vi "DB.vi"(0 "Data":T2={"Identity"=1, "Time"="俞忠达", "Meaning"="你好", "Thumb"=1, "Index"=1, "Middle"=1, "ring"=1, "little"=1, "wrist"=1, "arm"=1, "rota"=1, "delay"=1} {"arm" format="%#.0g"; "ring" format="%#.0g"; "Thumb" format="%#.0g"}, 1 "Beginning State":T5=enum."Inquire All DB" caption="状态", 2 "Delete Num":string[](array[string])=["0", "5"], 3 "Sort As":T3(ring)=enum."时间", 4 "Order":enum32{"Ascend", "Descend"}(radio), 5 "ErrI(No Error)":errorcluster, 6 "Data Table":T4={"Time_Table"="时间", "Meaning"="语义", "Thumb"="拇指", "arm"="手臂", "delay"="延时时间", "Identity"="ID", "passport"="", "Index"="食指", "Middle"="中指", "ring"="无名指", "little"="小手指", "wrist"="手腕", "rota"="转台", "Filename"="PZJData.mdb", "Table"="ACTION_DB"}, 7 "ID Manul？":bool) -> (13 "路径":string="Provider=Microsoft.Jet.OLEDB.4.0;Data Source=D:\\other\\项目\\手语项目\\Data Base\\PZJData.mdb;Persist Security Info=False", 14 "Data_Out":i32(listbox)=-1, 15 "Item Data":string[][](array[string])=[["0", "2017/2/3 20:41:53", "语义", "1", "1", "1", "1", "1", "1", "1", "1", "1"], ["1", "2017/2/3 20:43:36", "语义", "1", "1", "1", "1", "1", "1", "1", "1", "1"], ["2", "2017/2/3 20:51:23", "语义", "1", "1", "1", "1", "1", "1", "1", "1", "1"], ["3", "2017/2/3 20:51:25", "语义", "1", "1", "1", "1", "1", "1", "1", "1", "1"], ["4", "2017/2/3 20:51:26", "语义", "1", "1", "1", "1", "1", "1", "1", "1", "1"], ["5", "2017/2/3 20:51:27", "语义", "1", "1", "1", "1", "1", "1", "1", "1", "1"], ["6", "2017/2/3 20:51:29", "语义", "1", "1", "1", "1", "1", "1", "1", "1", "1"]], 16 "tables":string[](array[string])=["ACTION_DB"], 17 "State Out":string, 18 "New Data":string[](array[string]), 19 "ErrO":errorcluster)   [LabVIEW 2016]
uses:
  StateMachineStates.ctl
  Insertdata.ctl
  <vilib>/addons/database/Auxilliary.llb/DB Tools DataTypes.ctl
  <vilib>/addons/database/Connection.llb/DB Tools Open Connec (String).vi
  <vilib>/addons/database/Connection.llb/Conn Execute.vi
  <vilib>/addons/database/Recordset.llb/Rec Fetch Recordset Data (R).vi
  <vilib>/addons/database/Recordset.llb/Rec Destroy - Connection.vi
  <vilib>/addons/database/_DB Variant To Data/Database Variant To Data.xnode
  <vilib>/addons/database/NI_Database_API.lvlib
panel:
  out "输出簇":T1={"Identity"=6, "Time"="2017/2/3 20:51:29", "Meaning"="语义", "Thumb"=1, "Index"=1, "Middle"=1, "ring"=1, "little"=1, "wrist"=1, "arm"=1, "rota"=1, "delay"=1}
  out "Connection":string="Provider=Microsoft.Jet.OLEDB.4.0;Data Source=D:\\other\\项目\\手语项目\\Data Base\\PZJData.mdb;Persist Security Info=False"
  out "大小":i32[](array[numeric])=[3, 7]
  out "状态":bool
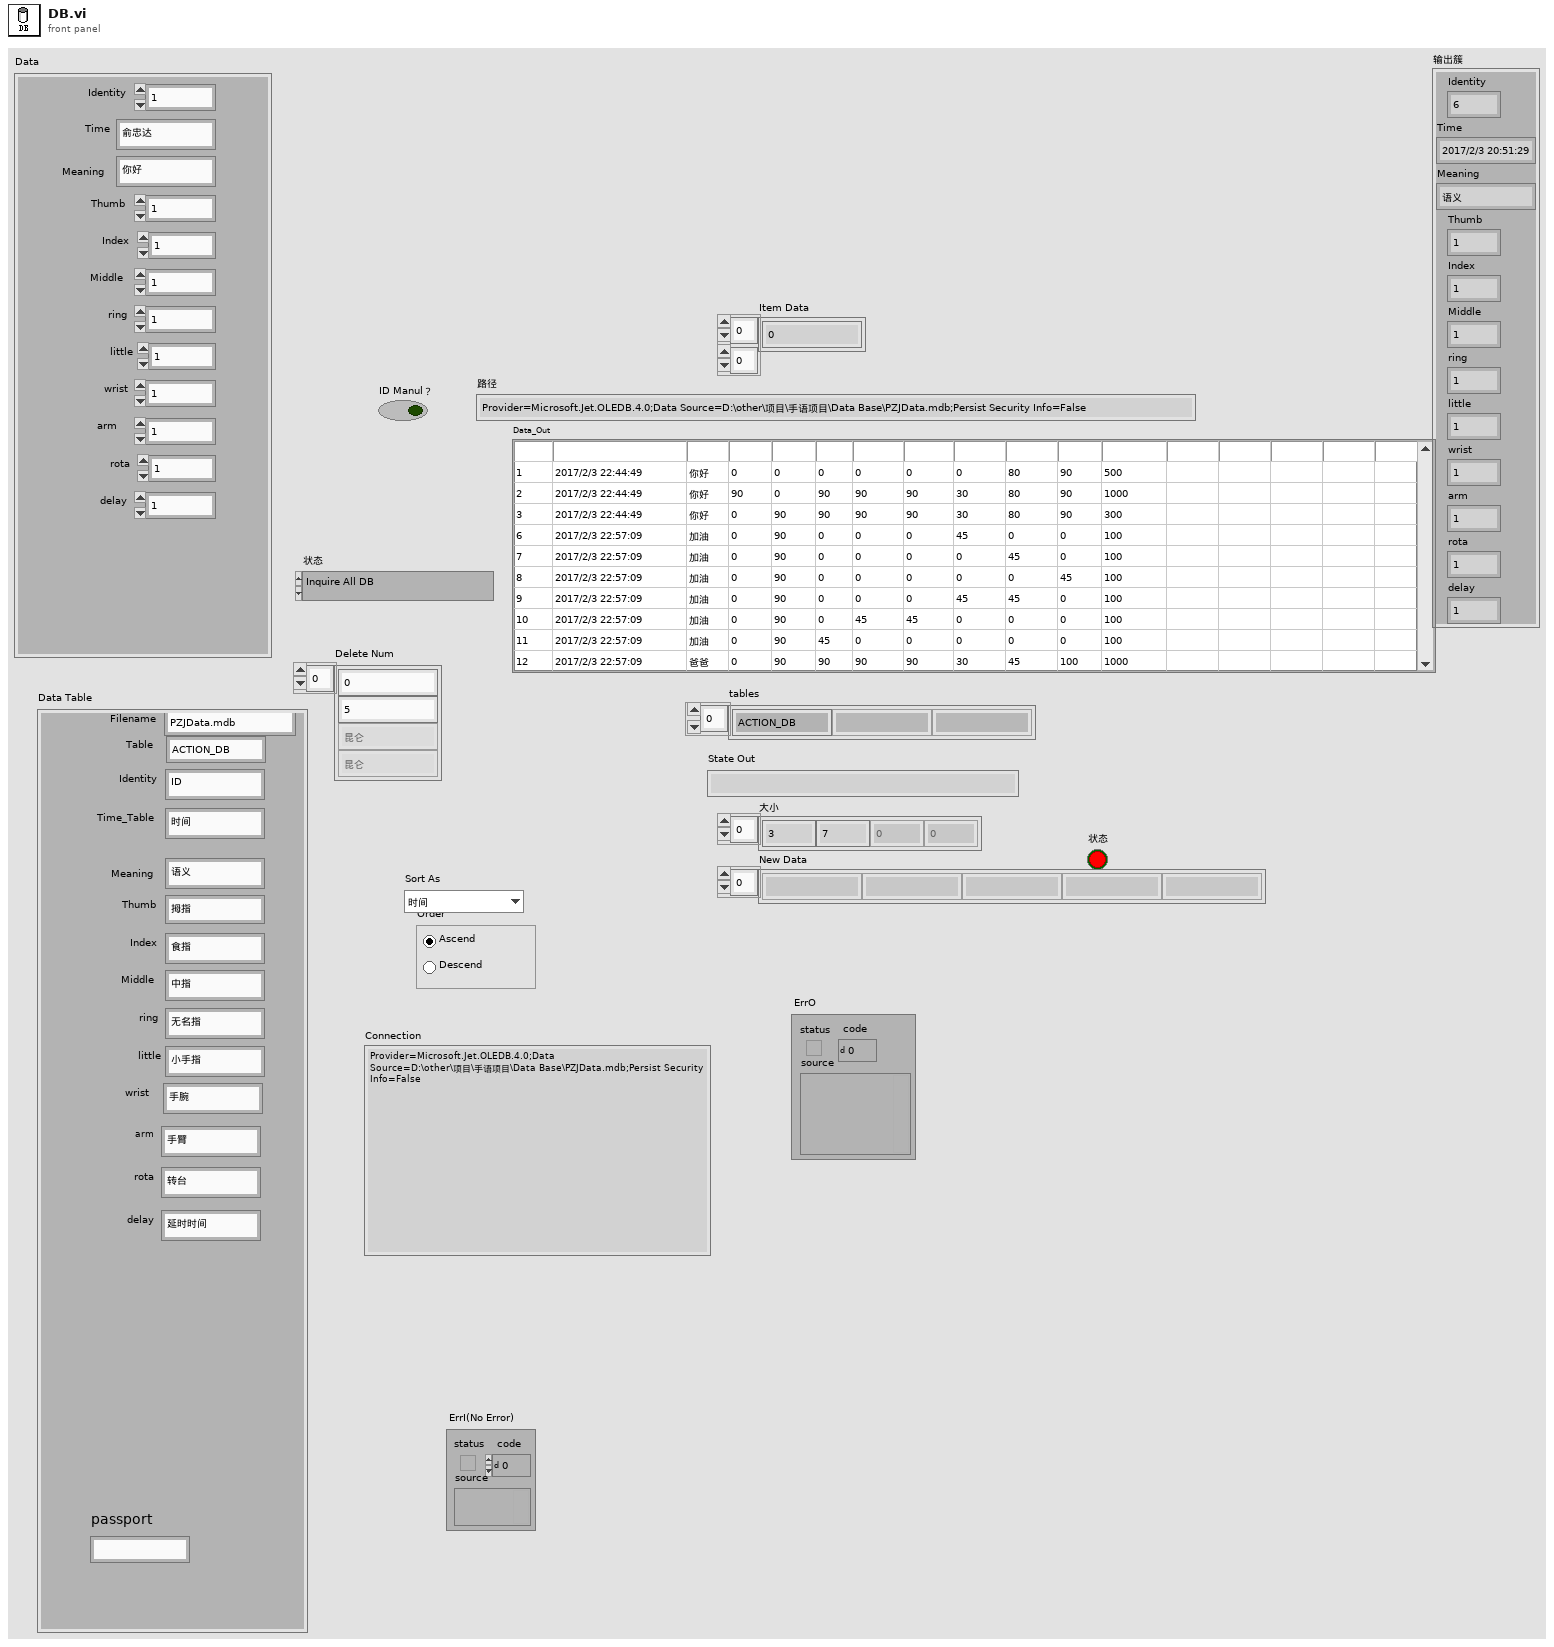
[diagram p1: front panel]
types:
  T1 = cluster{"Identity":i32, "Time":string, "Meaning":string, "Thumb":i32, "Index":i32, "Middle":i32, "ring":i32, "little":i32, "wrist":i32, "arm":i32, "rota":i32, "delay":i32}
  T2 = typedef "Insertdata.ctl" = cluster{"Identity":i32, "Time":string, "Meaning":string, "Thumb":i32, "Index":i32, "Middle":i32, "ring":i32, "little":i32, "wrist":i32, "arm":i32, "rota":i32, "delay":i32}
  T3 = enum16{"ID", "操作者", "级数", "个数", "角度", "时间", "机匣型号", ""}
  T4 = cluster{"Time_Table":string, "Meaning":string, "Thumb":string, "arm":string, "delay":string, "Identity":string, "passport":string, "Index":string, "Middle":string, "ring":string, "little":string, "wrist":string, "rota":string, "Filename":string, "Table":string}
  T5 = typedef "StateMachineStates.ctl" = enum16{"Connection DB", "Creat DB", "Delete Table", "Insert DB", "Inquire Table", "Inquire All DB", "Delete All Data", "Delete Data", "Sort Data", "Inquire Last Data", ""}
  T6 = typedef "NI_Database_API.lvlib/DB Tools DataTypes.ctl" = enum16{"String", "Long (I32)", "Single (SGL)", "Double (DBL)", "Date/Time", "Binary"}
  T7 = typedef "NI_Database_API.lvlib/DB Tools Column Info.ctl" = cluster{"column name":string, "data type":T6, "size":i32, "allow null?":bool}
  T8 = cluster{"Identity":dbl, "Time":string, "Operator":string, "Type":string, "Class":dbl, "Num":dbl, "Angle":dbl}
  T9 = typedef "NI_Database_API.lvlib/Conn ObjectReference.ctl" = refnum<k1>
  T10 = typedef "NI_Database_API.lvlib/Rec ObjectReference.ctl" = refnum<k1>
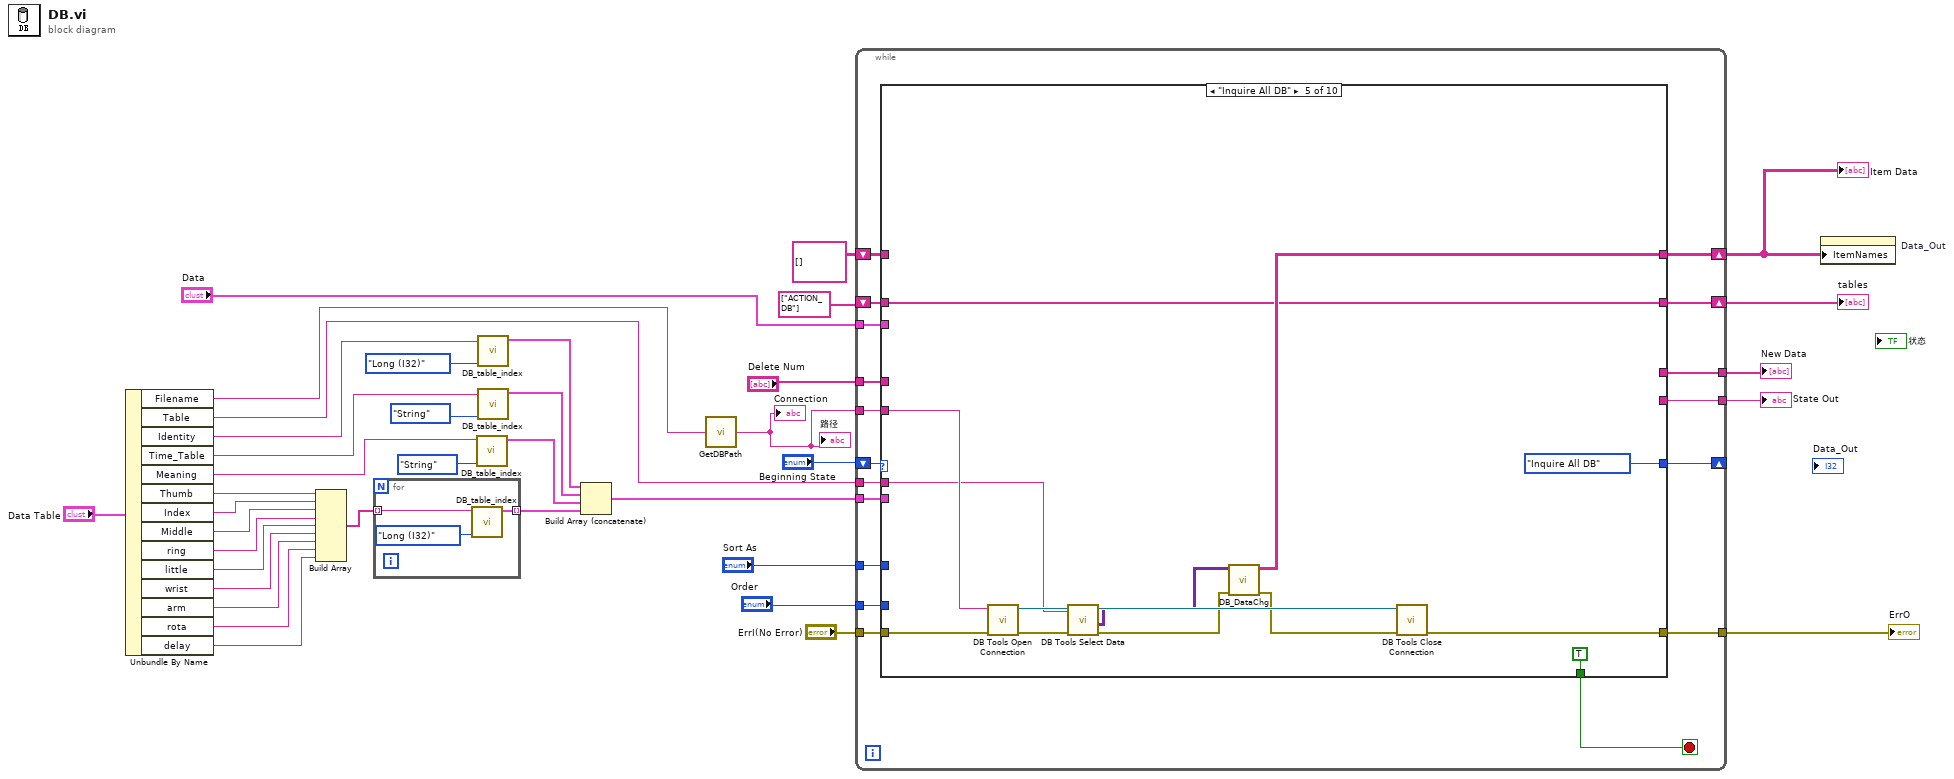
[diagram p0: block diagram]
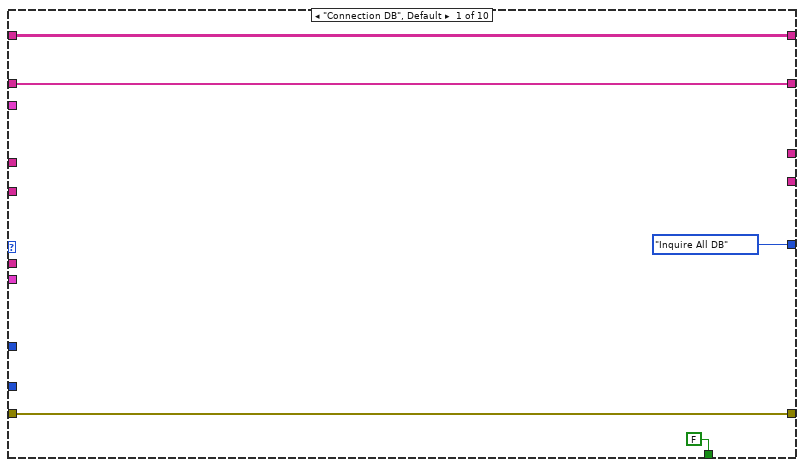
[diagram p2: hidden frame]
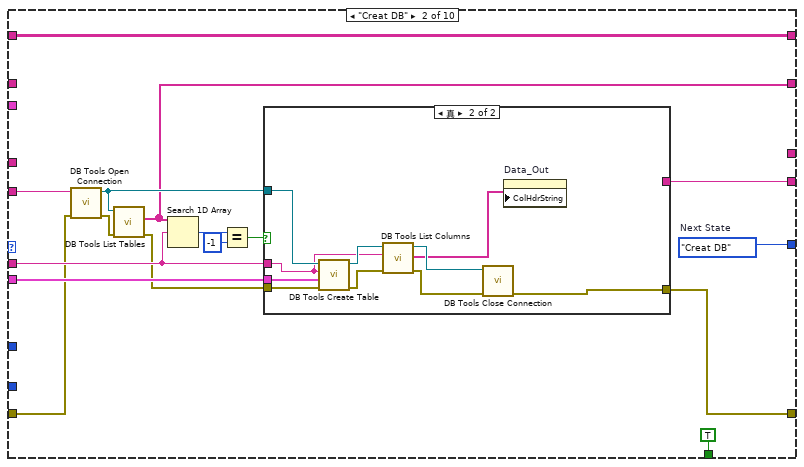
[diagram p3: hidden frame]
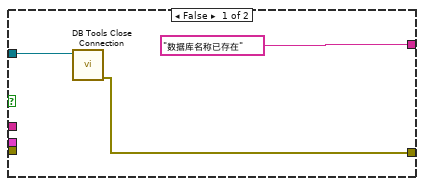
[diagram p4: hidden frame]
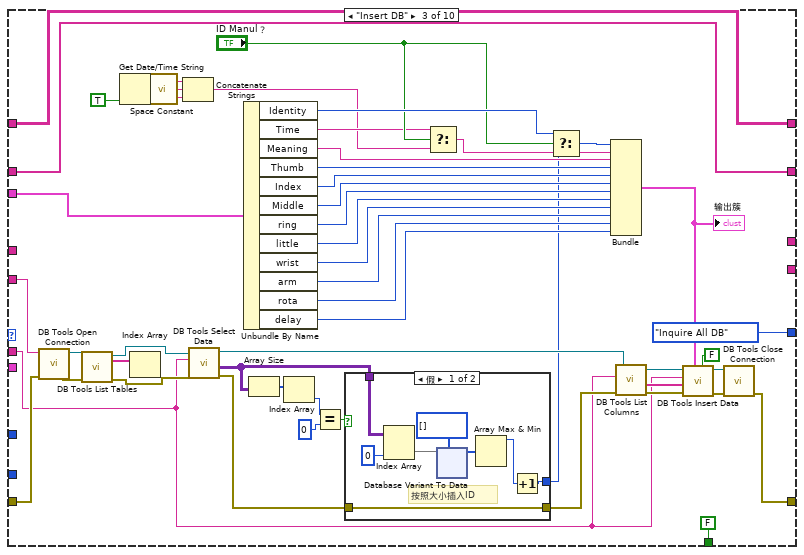
[diagram p5: hidden frame]
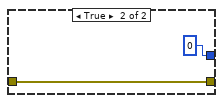
[diagram p6: hidden frame]
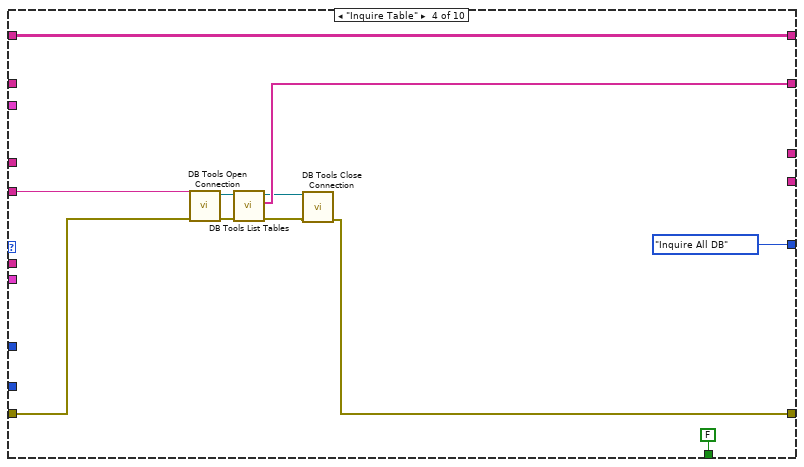
[diagram p7: hidden frame]
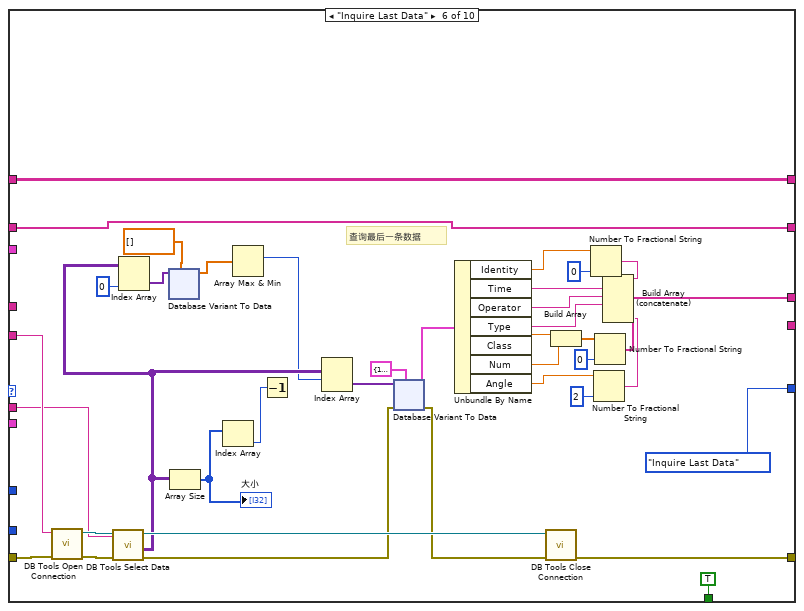
[diagram p8: hidden frame]
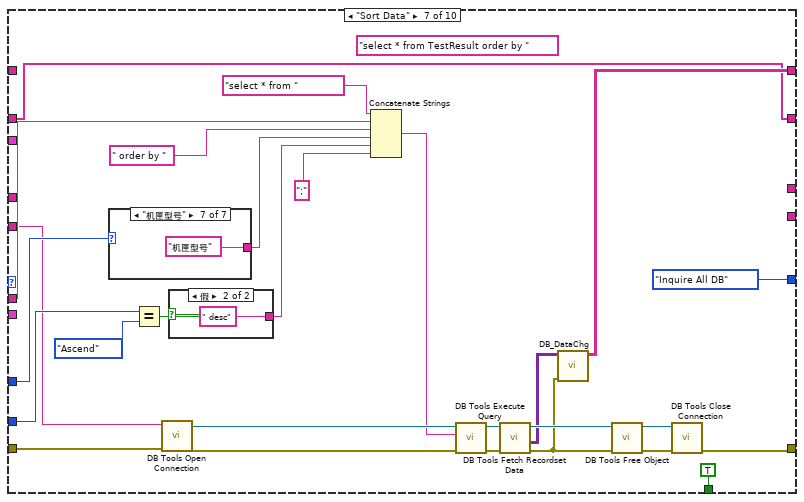
[diagram p9: hidden frame]
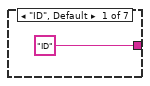
[diagram p10: hidden frame]
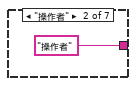
[diagram p11: hidden frame]
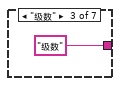
[diagram p12: hidden frame]
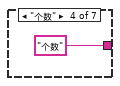
[diagram p13: hidden frame]
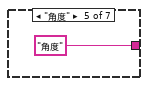
[diagram p14: hidden frame]
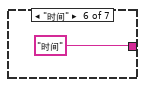
[diagram p15: hidden frame]
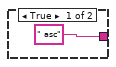
[diagram p16: hidden frame]
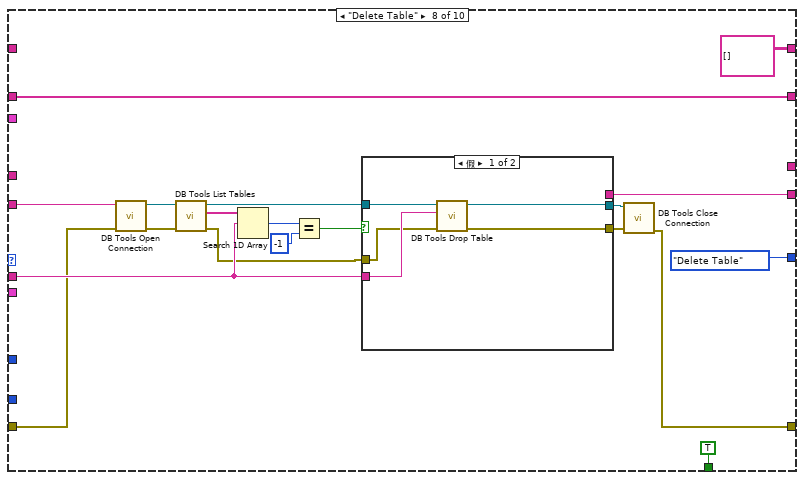
[diagram p17: hidden frame]
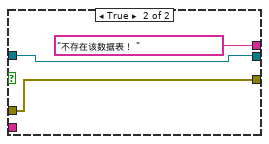
[diagram p18: hidden frame]
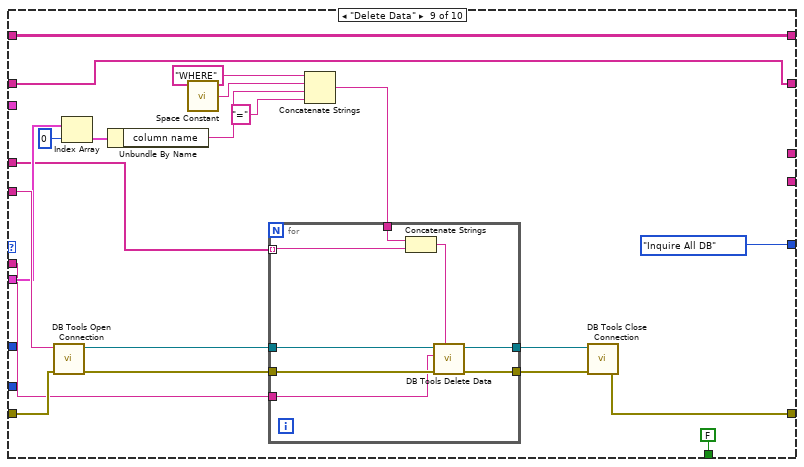
[diagram p19: hidden frame]
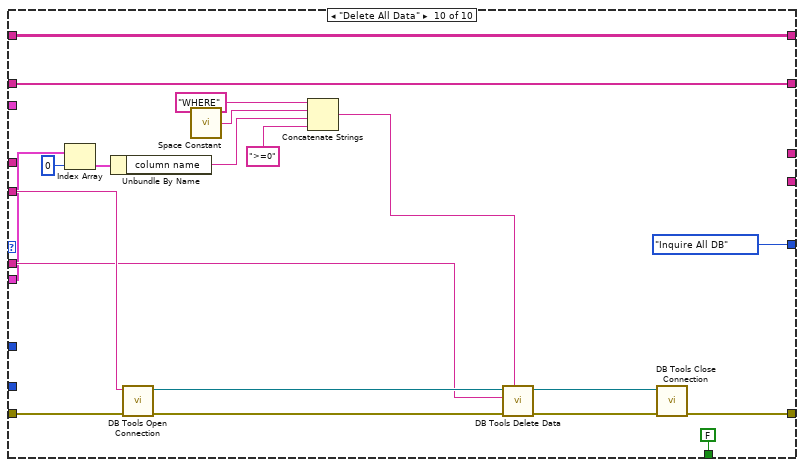
[diagram p20: hidden frame]
diagram:
  n1 = Unbundle By Name("Data Table") -> ("Filename"=w25:string, "Table"=w24:string, "Identity"=w21:string, "Time_Table"=w18:string, "Meaning"=w15:string, "Thumb"=w10:string, "Index"=w9:string, "Middle"=w8:string, "ring"=w7:string, "little"=w6:string, "wrist"=w5:string, "arm"=w4:string, "rota"=w3:string, "delay"=w2:string)
  n2 = Build Array(w10, w9, w8, w7, w6, w5, w4, w3, w2) -> (w1:string[])
  n3 = for {
    tunnel: [w41] -> w36 mode=indexing
    tunnel: w1 -> [w39] mode=indexing
    n4 = call "DB_table_index.vi"("data type"=DB_Tools_DataTypes."Long (I32)", "Thumb"=w39) -> ("column information 2"=w41:T7)  [unwired: 9 in]
  }
  n5 = call "DB_table_index.vi"("data type"=DB_Tools_DataTypes."String", "Thumb"=w15) -> ("column information 2"=w14:T7)  [unwired: 9 in]
  n6 = call "DB_table_index.vi"("data type"=DB_Tools_DataTypes."Long (I32)", "Thumb"=w21) -> ("column information 2"=w20:T7)  [unwired: 9 in]
  n7 = call "DB_table_index.vi"("data type"=DB_Tools_DataTypes."String", "Thumb"=w18) -> ("column information 2"=w16:T7)  [unwired: 9 in]
  n8 = Build Array (concatenate)(w20, w16, w14, w36) -> (w37:T7[])
  n9 = call "GetDBPath.vi"("Filename"=w25) -> ("Connection"=w23:string)
  "Connection" <- w23
  "路径" <- w23
  n10 = while {
    shift-right: [w58] -> _
    shift-left: "Beginning State" -> [w59]
    tunnel: w37 -> [w57]
    tunnel: w24 -> [w56]
    tunnel: w23 -> [w55]
    tunnel: [w54] -> w35
    tunnel: "ErrI(No Error)" -> [w52]
    tunnel: [w51] -> w32
    tunnel: "Data" -> [w50]
    shift-right: [w49] -> w30
    shift-left: string[][] [] -> [w48]
    tunnel: "Delete Num" -> [w46]
    tunnel: "Sort As" -> [w45]
    tunnel: "Order" -> [w44]
    tunnel: [w43] -> w22
    shift-right: [w53] -> w34
    shift-left: string[] ["ACTION_DB"] ("tables 2") -> [w42]
    stop <- w47 stop-if-true
    n11 = case shown="\"Inquire All DB\"" w59 {
      tunnel: [StateMachineStates."Inquire All DB" ("Next State") w80 StateMachineStates."Inquire All DB" ("Next State") StateMachineStates."Inquire All DB" ("Next State") StateMachineStates."Inquire All DB" ("Next State") StateMachineStates."Inquire Last Data" ("Next State") StateMachineStates."Inquire All DB" ("Next State") StateMachineStates."Delete Table" ("Next State") StateMachineStates."Inquire All DB" ("Next State") StateMachineStates."Inquire All DB" ("Next State")] -> w58
      tunnel: w57 -> [_ w73 _ _ _ _ _ _ w594 w609]
      tunnel: w56 -> [_ w72 w94 _ w212 w251 w531 w562 w587 w619]
      tunnel: w55 -> [_ w79 w143 w201 w216 w252 w521 w568 w596 w622]
      tunnel: [_ w74 _ _ _ _ _ w560 _ _] -> w54
      tunnel: [w60 w71 w96 w198 w203 w217 w515 w551 w578 w607] -> w53
      tunnel: w52 -> [w64 w66 w142 w200 w215 w228 w523 w554 w595 w623]
      tunnel: [w64 w70 w136 w195 w210 w248 w522 w555 w582 w616] -> w51
      tunnel: w50 -> [_ _ w109 _ _ _ _ _ _ _]
      tunnel: [w63 w69 w108 w194 w208 w247 w516 string[][] [] w579 w624] -> w49
      tunnel: w48 -> [w63 w69 w108 w194 _ w247 _ _ w579 w624]
      tunnel: [FALSE TRUE FALSE FALSE TRUE TRUE TRUE TRUE FALSE FALSE] -> w47
      tunnel: w46 -> [_ _ _ _ _ _ _ _ w580 _]
      tunnel: w45 -> [_ _ _ _ _ _ w535 _ _ _]
      tunnel: w44 -> [_ _ _ _ _ _ w534 _ _ _]
      tunnel: [_ _ _ _ _ w219 _ _ _ _] -> w43
      tunnel: w42 -> [w60 _ w96 _ w203 w217 w515 w551 w578 w607]
      frame "Connection DB", Default {
      }
      frame "Creat DB" {
        w80 = StateMachineStates."Creat DB"  # Next State
        n12 = call-poly <vilib>:"DB Tools Open Connection.vi"("error in (no error)"=w66, "connection information"=w79) -> ("error out"=w67:errorcluster, "connection reference"=w78:T9)  [unwired: 6 in]
        n13 = call <vilib>:"DB Tools List Tables.vi"("error in (no error)"=w67, "connection reference"=w78) -> ("error out"=w65:errorcluster, "tables"=w71:string[])  [unwired: 3 in, 1 out]
        n14 = Search 1D Array(1D array=w71, element=w72) -> (index of element=w77:i32)  [unwired: 1 in]
        n15 = Equal?(x=w77, y=-1) -> (x = y?=w75:bool)
        n16 = case shown="真" w75 {
          tunnel: w78 -> [w82 w93]
          tunnel: ["数据库名称已存在" _] -> w74
          tunnel: w73 -> [_ w92]
          tunnel: w72 -> [_ w87]
          tunnel: [w81 w91] -> w70
          tunnel: w65 -> [_ w90]
          frame False {
            n17 = call <vilib>:"DB Tools Close Connection.vi"("connection reference"=w82) -> ("error out"=w81:errorcluster)  [unwired: 6 in]
          }
          frame True {
            n18 = call <vilib>:"DB Tools Create Table.vi"("error in (no error)"=w90, "column information"=w92, "table"=w87, "connection reference"=w93) -> ("error out"=w85:errorcluster, "connection reference out"=w89:T9)  [unwired: 4 in]
            n19 = call <vilib>:"DB Tools List Columns.vi"("error in (no error)"=w85, "table"=w87, "connection reference"=w89) -> ("error out"=w84:errorcluster, "columns"=w86:string[], "connection reference out"=w88:T9)  [unwired: 1 in, 1 out]
            n20 = call <vilib>:"DB Tools Close Connection.vi"("error in (no error)"=w84, "connection reference"=w88) -> ("error out"=w91:errorcluster)  [unwired: 5 in]
            n21 = property on="Data_Out" class="MCListbox (严格)"("ColHdrString"=w86) -> ()  [unwired: 2 in, 2 out]
          }
        }
      }
      frame "Insert DB" {
        n22 = call-poly <vilib>:"DB Tools Open Connection.vi"("error in (no error)"=w142, "connection information"=w143) -> ("error out"=w101:errorcluster, "connection reference"=w95:T9)  [unwired: 6 in]
        n23 = call <vilib>:"DB Tools List Tables.vi"("error in (no error)"=w101, "connection reference"=w95) -> ("error out"=w99:errorcluster, "tables"=w100:string[], "connection reference out"=w98:T9)  [unwired: 3 in]
        n24 = Get Date/Time String(want seconds? (F)=TRUE) -> (date string=w115:string, time string=w117:string)  [unwired: 2 in]
        n25 = Index Array(array=w100) -> ()  [unwired: 1 in, 1 out]
        n26 = call <vilib>:"Space Constant.vi"() -> ("String"=w116:string)
        n27 = Concatenate Strings(w115, w116, w117) -> (w111:string)
        n28 = call <vilib>:"DB Tools Select Data.vi"("error in (no error)"=w99, "table"=w94, "connection reference"=w98) -> ("error out"=w132:errorcluster, "data"=w120:variant[][], "connection reference out"=w134:T9)  [unwired: 3 in]
        n29 = Unbundle By Name(w109) -> ("Identity"=w118:i32, "Time"=w112:string, "Meaning"=w127:string, "Thumb"=w128:i32, "Index"=w129:i32, "Middle"=w130:i32, "ring"=w131:i32, "little"=w107:i32, "wrist"=w106:i32, "arm"=w105:i32, "rota"=w104:i32, "delay"=w103:i32)
        n30 = Array Size(array=w120) -> (size(s)=w126:i32[])
        n31 = Index Array(array=w126) -> (element=w123:i32)  [unwired: 1 in]
        n32 = Equal?(x=w123, y=0) -> (x = y?=w124:bool)
        n33 = case shown="假" w124 {
          tunnel: [w146 w191] -> w133
          tunnel: w132 -> [w146 w191]
          tunnel: w120 -> [w151 _]
          tunnel: [w144 0] -> w102
          frame False {
            # "按照大小插入ID"
            n34 = Index Array(array=w151, index (col)=0 ("索引 (行)")) -> (element=w149:variant[])  [unwired: 1 in]
            n35 = xnode "Database Variant To Data"("database variant"=w149, "type"=i32[] []) -> ("data"=w147:i32[])  [unwired: 1 in, 1 out]
            n36 = Array Max & Min(array=w147) -> (max value=w145:i32)  [unwired: 3 out]
            n37 = Increment(x=w145) -> (x+1=w144:i32)
          }
          frame True {
          }
        }
        n38 = Select(t=w112, s="ID Manul？", f=w111) -> (s? t:f=w110:string)
        n39 = Select(t=w118, s="ID Manul？", f=w102) -> (s? t:f=w119:i32)
        n40 = Bundle("Identity"=w119, "Time"=w110, "Meaning"=w127, "Thumb"=w128, "Index"=w129, "Middle"=w130, "ring"=w131, "little"=w107, "wrist"=w106, "arm"=w105, "rota"=w104, "delay"=w103) -> (w97:T1)  [unwired: 1 in]
        "输出簇" <- w97
        n41 = call <vilib>:"DB Tools List Columns.vi"("error in (no error)"=w133, "table"=w94, "connection reference"=w134) -> ("error out"=w141:errorcluster, "columns"=w140:string[], "connection reference out"=w137:T9)  [unwired: 1 in, 1 out]
        n42 = call <vilib>:"DB Tools Insert Data.vi"("create table? (F)"=FALSE, "data"=w97, "error in (no error)"=w141, "columns"=w140, "table"=w94, "connection reference"=w137) -> ("error out"=w138:errorcluster, "connection reference out"=w139:T9)  [unwired: 4 in]
        n43 = call <vilib>:"DB Tools Close Connection.vi"("error in (no error)"=w138, "connection reference"=w139) -> ("error out"=w136:errorcluster)  [unwired: 5 in]
      }
      frame "Inquire Table" {
        n44 = call-poly <vilib>:"DB Tools Open Connection.vi"("error in (no error)"=w200, "connection information"=w201) -> ("error out"=w199:errorcluster, "connection reference"=w202:T9)  [unwired: 6 in]
        n45 = call <vilib>:"DB Tools List Tables.vi"("error in (no error)"=w199, "connection reference"=w202) -> ("error out"=w196:errorcluster, "tables"=w198:string[], "connection reference out"=w197:T9)  [unwired: 3 in]
        n46 = call <vilib>:"DB Tools Close Connection.vi"("error in (no error)"=w196, "connection reference"=w197) -> ("error out"=w195:errorcluster)  [unwired: 5 in]
      }
      frame "Inquire All DB" {
        n47 = call-poly <vilib>:"DB Tools Open Connection.vi"("error in (no error)"=w215, "connection information"=w216) -> ("error out"=w213:errorcluster, "connection reference"=w214:T9)  [unwired: 6 in]
        n48 = call <vilib>:"DB Tools Select Data.vi"("error in (no error)"=w213, "table"=w212, "connection reference"=w214) -> ("error out"=w207:errorcluster, "data"=w209:variant[][], "connection reference out"=w211:T9)  [unwired: 3 in]
        n49 = call "DB_DataChg.vi"("错误输入（无错误）"=w207, "data"=w209) -> ("错误输出"=w206:errorcluster, "数组"=w208:string[][])  [unwired: 8 in]
        n50 = call <vilib>:"DB Tools Close Connection.vi"("error in (no error)"=w206, "connection reference"=w211) -> ("error out"=w210:errorcluster)  [unwired: 5 in]
      }
      frame "Inquire Last Data" {
        # "查询最后一条数据"
        n51 = call-poly <vilib>:"DB Tools Open Connection.vi"("error in (no error)"=w228, "connection information"=w252) -> ("error out"=w254:errorcluster, "connection reference"=w255:T9)  [unwired: 6 in]
        n52 = call <vilib>:"DB Tools Select Data.vi"("error in (no error)"=w254, "table"=w251, "connection reference"=w255) -> ("error out"=w226:errorcluster, "data"=w221:variant[][], "connection reference out"=w253:T9)  [unwired: 3 in]
        n53 = Index Array(array=w221, index (col)=0 ("索引 (行)")) -> (element=w223:variant[])  [unwired: 1 in]
        n54 = xnode "Database Variant To Data"("database variant"=w223, "type"=dbl[] []) -> ("data"=w222:dbl[])  [unwired: 1 in, 1 out]
        n55 = Array Size(array=w221) -> (size(s)=w246:i32[])
        "大小" <- w246
        n56 = Index Array(array=w246) -> (element=w245:i32)  [unwired: 1 in]
        n57 = Array Max & Min(array=w222) -> (max index (indices)=w218:i32)  [unwired: 3 out]
        n58 = Decrement(x=w245) -> ()  [unwired: 1 out]
        n59 = Index Array(array=w221, index (row)=w218) -> (element=w227:variant[])  [unwired: 1 in]
        n60 = xnode "Database Variant To Data"("database variant"=w227, "error in (no error)"=w226, "type"=T8 {"Identity"=1.0, "Time"="", "Operator"="俞忠达", "Type"="WS11", "Class"=1.23, "Num"=1.23, "Angle"=1.23}) -> ("data"=w244:T8, "error out"=w225:errorcluster)
        n61 = Unbundle By Name(w244) -> ("Identity"=w236:dbl, "Time"=w240:string, "Operator"=w239:string, "Type"=w238:string, "Class"=w242:dbl, "Num"=w243:dbl, "Angle"=w232:dbl)
        n62 = call <vilib>:"DB Tools Close Connection.vi"("error in (no error)"=w225, "connection reference"=w253) -> ("error out"=w248:errorcluster)  [unwired: 5 in]
        n63 = Build Array(w242, w243) -> (w241:dbl[])
        n64 = Number To Fractional String(number=w236, precision (6)=i16 0 ("精度(6)")) -> (F-format string=w235:string)  [unwired: 2 in]
        n65 = Number To Fractional String(number=w232, precision (6)=i16 2 ("精度(6)")) -> (F-format string=w230:string)  [unwired: 2 in]
        n66 = Number To Fractional String(number=w241, precision (6)=i16 0 ("精度(6)")) -> (F-format string=w237:string[])  [unwired: 2 in]
        n67 = Build Array (concatenate)(w235, w240, w239, w238, w237, w230) -> (w219:string[])
      }
      frame "Sort Data" {
        (unwired) "select * from TestResult order by " ("SQL query")
        n68 = case shown="\"机匣型号\"" w535 {
          tunnel: ["ID" "操作者" "级数" "个数" "角度" "时间" "机匣型号"] -> w537
          frame "ID", Default {
          }
          frame "操作者" {
          }
          frame "级数" {
          }
          frame "个数" {
          }
          frame "角度" {
          }
          frame "时间" {
          }
          frame "机匣型号" {
          }
        }
        n69 = Equal?(x=w534, y=enum32{"Ascend", "Descend"}."Ascend" ("Order")) -> (x = y?=w541:bool)
        n70 = call-poly <vilib>:"DB Tools Open Connection.vi"("error in (no error)"=w523, "connection information"=w521) -> ("error out"=w525:errorcluster, "connection reference"=w524:T9)  [unwired: 6 in]
        n71 = case shown="假" w541 {
          tunnel: [" asc" ("Substring") " desc" ("Substring")] -> w539
          frame True {
          }
          frame False {
          }
        }
        n72 = Concatenate Strings("select * from " ("SQL query"), w531, " order by " ("SQL query"), w537, w539, ";" ("Substring")) -> (w520:string)
        n73 = call-poly <vilib>:"DB Tools Execute Query.vi"("error in (no error)"=w525, "SQL query"=w520, "connection reference"=w524) -> ("error out"=w527:errorcluster, "recordset reference"=w526:T10)  [unwired: 5 in]
        n74 = call-poly <vilib>:"DB Tools Fetch Recordset Data.vi"("error in (no error)"=w527, "recordset reference"=w526) -> ("error out"=w518:errorcluster, "recordset data"=w517:variant[][], "recordset reference out"=w528:T10)  [unwired: 3 in]
        n75 = call "DB_DataChg.vi"("错误输入（无错误）"=w518, "data"=w517) -> ("数组"=w516:string[][])  [unwired: 8 in, 1 out]
        n76 = call-poly <vilib>:"DB Tools Free Object.vi"("error in (no error)"=w518, "recordset reference"=w528) -> ("error out"=w530:errorcluster, "connection reference"=w529:T9)  [unwired: 8 in]
        n77 = call <vilib>:"DB Tools Close Connection.vi"("error in (no error)"=w530, "connection reference"=w529) -> ("error out"=w522:errorcluster)  [unwired: 5 in]
      }
      frame "Delete Table" {
        n78 = call-poly <vilib>:"DB Tools Open Connection.vi"("error in (no error)"=w554, "connection information"=w568) -> ("error out"=w564:errorcluster, "connection reference"=w565:T9)  [unwired: 6 in]
        n79 = call <vilib>:"DB Tools List Tables.vi"("error in (no error)"=w564, "connection reference"=w565) -> ("error out"=w556:errorcluster, "tables"=w563:string[], "connection reference out"=w559:T9)  [unwired: 3 in]
        n80 = Search 1D Array(1D array=w563, element=w562) -> (index of element=w567:i32)  [unwired: 1 in]
        n81 = Equal?(x=w567, y=-1) -> (x = y?=w561:bool)
        n82 = case shown="假" w561 {
          tunnel: w562 -> [w574 _]
          tunnel: [_ "不存在该数据表！ "] -> w560
          tunnel: w559 -> [w573 w575]
          tunnel: [w572 w575] -> w558
          tunnel: [w571 w576] -> w557
          tunnel: w556 -> [w570 w576]
          frame False {
            n83 = call <vilib>:"DB Tools Drop Table.vi"("error in (no error)"=w570, "table"=w574, "connection reference"=w573) -> ("error out"=w571:errorcluster, "connection reference out"=w572:T9)  [unwired: 5 in]
          }
          frame True {
          }
        }
        n84 = call <vilib>:"DB Tools Close Connection.vi"("error in (no error)"=w557, "connection reference"=w558) -> ("error out"=w555:errorcluster)  [unwired: 5 in]
      }
      frame "Delete Data" {
        n85 = call-poly <vilib>:"DB Tools Open Connection.vi"("error in (no error)"=w595, "connection information"=w596) -> ("error out"=w590:errorcluster, "connection reference"=w591:T9)  [unwired: 6 in]
        n86 = Index Array(array=w594, index=0 ("索引")) -> (element=w592:T7)
        n87 = Unbundle By Name(w592) -> ("column name"=w584:string)
        n88 = call <vilib>:"Space Constant.vi"() -> ("String"=w585:string)
        n89 = Concatenate Strings("WHERE" ("delete optional clause"), w585, w584, "=") -> (w581:string)
        n90 = for {
          tunnel: w591 -> [w606]
          tunnel: w590 -> [w605]
          tunnel: [w604] -> w589
          tunnel: [w603] -> w588
          tunnel: w587 -> [w602]
          tunnel: w581 -> [w599]
          tunnel: w580 -> [w601] mode=indexing
          n91 = Concatenate Strings(w599, w601) -> (w600:string)
          n92 = call <vilib>:"DB Tools Delete Data.vi"("condition"=w600, "error in (no error)"=w605, "table"=w602, "connection reference"=w606) -> ("error out"=w604:errorcluster, "connection reference out"=w603:T9)  [unwired: 6 in]
        }
        n93 = call <vilib>:"DB Tools Close Connection.vi"("error in (no error)"=w589, "connection reference"=w588) -> ("error out"=w582:errorcluster)  [unwired: 5 in]
      }
      frame "Delete All Data" {
        n94 = Index Array(array=w609, index=0 ("索引")) -> (element=w614:T7)
        n95 = Unbundle By Name(w614) -> ("column name"=w611:string)
        n96 = call-poly <vilib>:"DB Tools Open Connection.vi"("error in (no error)"=w623, "connection information"=w622) -> ("error out"=w620:errorcluster, "connection reference"=w621:T9)  [unwired: 6 in]
        n97 = call <vilib>:"Space Constant.vi"() -> ("String"=w612:string)
        n98 = Concatenate Strings("WHERE" ("delete optional clause"), w612, w611, ">=0") -> (w608:string)
        n99 = call <vilib>:"DB Tools Delete Data.vi"("condition"=w608, "error in (no error)"=w620, "table"=w619, "connection reference"=w621) -> ("error out"=w617:errorcluster, "connection reference out"=w618:T9)  [unwired: 6 in]
        n100 = call <vilib>:"DB Tools Close Connection.vi"("error in (no error)"=w617, "connection reference"=w618) -> ("error out"=w616:errorcluster)  [unwired: 5 in]
      }
    }
  }
  "State Out" <- w35
  "tables" <- w34
  "ErrO" <- w32
  "Item Data" <- w30
  "New Data" <- w22
  n101 = property on="Data_Out" class="MCListbox (严格)"("ItemNames"=w30) -> ()  [unwired: 2 in, 2 out]
